vi "Label Targets AprilTagl.vi"(5 "Details":bool, 7 "Annotate":bool=TRUE, 9 "results":T1={"diameter points"={"first point"={"x"=0.0, "y"=0.0}, "projected point"={"x"=0.0, "y"=0.0}}, "normalized center"={"x"=0.0, "y"=0.0}, "Overall Score"=0.0, "Distance (ft)"=0.0, "Offset Angle"=0.0, "Tag corner points"=[], "Tag Center"={"X"=0.0, "Y"=0.0}, "Tag Yaw"=0.0, "Tag Pitch"=0.0, "Target Roll (deg)"=0.0, "AprilTag Number"=68} {"Tag Center"."Y" format="%0.2f"; "Tag Center"."X" format="%0.2f"}, 10 "Angle":dbl=53.2 format="%#_13g", 11 "Image in":T2) -> (3 "Image out":T2)   [LabVIEW 2023]
doc: "Draw scores near or on the particle and an ellipse around the target. Scores that are below the score threshold are drawn in red, above in green."
uses:
  <vilib>/vision/Image Controls.llb/IMAQ Image.ctl
  AprilTag Target Fields.ctl
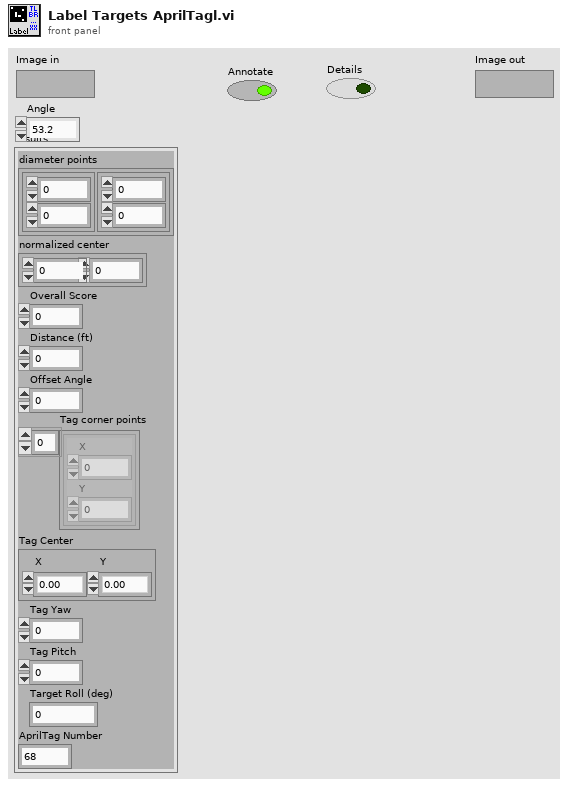
[diagram p1: front panel]
types:
  T1 = typedef "AprilTag Target Fields.ctl" = cluster{"diameter points":cluster{"first point":cluster{"x":dbl, "y":dbl}, "projected point":cluster{"x":dbl, "y":dbl}}, "normalized center":cluster{"x":dbl, "y":dbl}, "Overall Score":dbl, "Distance (ft)":dbl, "Offset Angle":dbl, "Tag corner points":cluster{"X":dbl, "Y":dbl}[], "Tag Center":cluster{"X":dbl, "Y":dbl}, "Tag Yaw":dbl, "Tag Pitch":dbl, "Target Roll (deg)":dbl, "AprilTag Number":i32}
  T2 = typedef "IMAQ Image.ctl" = refnum<image>
  T3 = cluster{"Desired Font (Application)":enum16{"User-specified Font", "Application Font", "System Font", "Dialog Font"}, "[User-specified Font]":cluster{"Font Name":string, "Size":i16, "Strikeout?":bool, "Italic?":bool, "Underline?":bool, "Outline?":bool, "Shadow?":bool, "Bold?":bool, "Rotation Angle":dbl}, "Horizontal Alignment":i16, "Vertical Alignment":i16}
  T4 = cluster{"first point":cluster{"x":dbl, "y":dbl}, "projected point":cluster{"x":dbl, "y":dbl}}
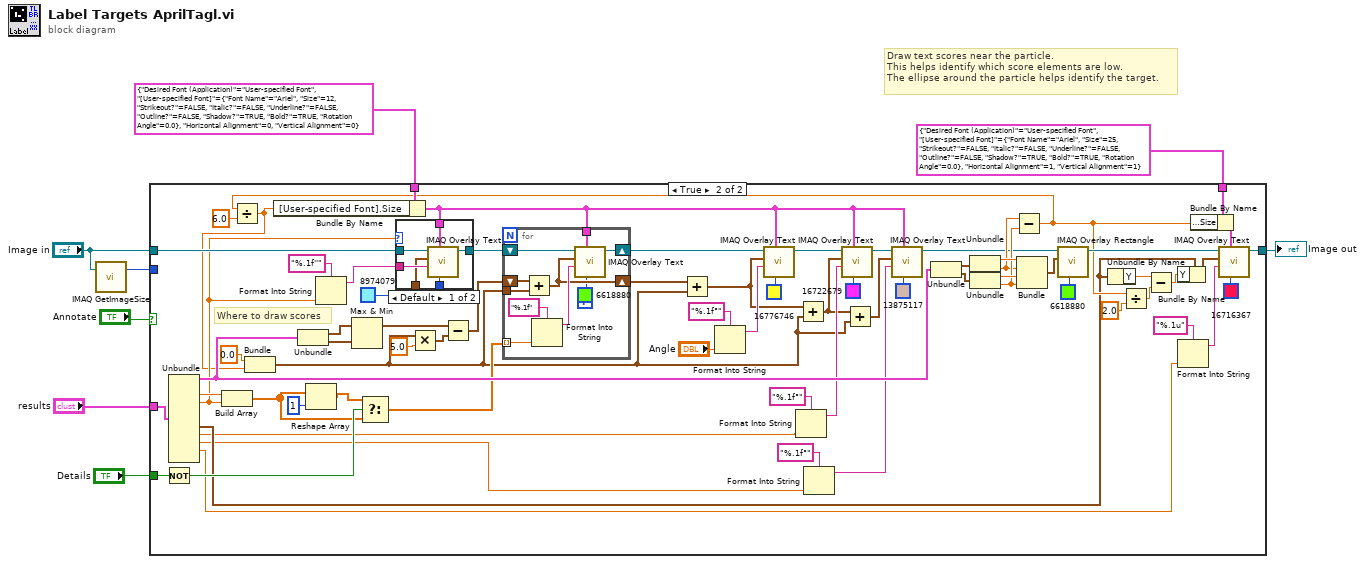
[diagram p0: block diagram]
diagram:
  # "Draw text scores near the particle.\nThis helps identify which score elements are low.\nThe ellipse around the particle helps identify the target."
  n1 = call "IMAQ GetImageSize"("Image"="Image in") -> ("Y Resolution"=w6:i32)  [unwired: 3 in, 2 out]
  n2 = case shown="True" "Annotate" {
    tunnel: [w9 w40] -> w8
    tunnel: "Image in" -> [w9 w79]
    tunnel: w6 -> [_ _]
    tunnel: "results" -> [_ w75]
    tunnel: "Details" -> [_ w66]
    tunnel: T3 {"Desired Font (Application)"=enum."User-specified Font", "[User-specified Font]"={"Font Name"="Ariel", "Size"=25, "Strikeout?"=FALSE, "Italic?"=FALSE, "Underline?"=FALSE, "Outline?"=FALSE, "Shadow?"=TRUE, "Bold?"=TRUE, "Rotation Angle"=0.0}, "Horizontal Alignment"=1, "Vertical Alignment"=1} ("Font, Size & Style") -> [_ w44]
    tunnel: T3 {"Desired Font (Application)"=enum."User-specified Font", "[User-specified Font]"={"Font Name"="Ariel", "Size"=12, "Strikeout?"=FALSE, "Italic?"=FALSE, "Underline?"=FALSE, "Outline?"=FALSE, "Shadow?"=TRUE, "Bold?"=TRUE, "Rotation Angle"=0.0}, "Horizontal Alignment"=0, "Vertical Alignment"=0} ("Font, Size & Style") -> [_ w26]
    frame False {
    }
    frame True {
      # "Where to draw scores"
      n3 = Not(x=w66) -> (.not. x?=w65:bool)
      n4 = Unbundle(w75) -> ("diameter points"=w70:T4, "Overall Score"=w59:dbl, "Distance (ft)"=w32:dbl, "Tag Center"=w13:cluster{"X":dbl, "Y":dbl}, "Tag Yaw"=w12:dbl, "Tag Pitch"=w11:dbl, "Target Roll (deg)"=w10:dbl)  [unwired: 4 out]
      n5 = Build Array(w59, w32) -> (w63:dbl[])
      n6 = Unbundle(w70) -> ("first point"=w72:cluster{"x":dbl, "y":dbl}, "projected point"=w73:cluster{"x":dbl, "y":dbl})
      n7 = Reshape Array(w63, 1) -> (w64:dbl[])
      n8 = Format Into String(format string="%.1f''", w32) -> (resulting string=w78:string)  [unwired: 2 in, 1 out]
      n9 = Max & Min(x=w72, y=w73) -> (max(x,y)=w51:cluster{"x":dbl, "y":dbl})  [unwired: 1 out]
      n10 = Select(t=w64, s=w65, f=w63) -> (s? t:f=w62:dbl[])
      n11 = Format Into String(format string="%.1f°", "Angle") -> (resulting string=w57:string)  [unwired: 2 in, 1 out]
      n12 = Format Into String(format string="%.1f°", w12) -> (resulting string=w31:string)  [unwired: 2 in, 1 out]
      n13 = Format Into String(format string="%.1f°", w11) -> (resulting string=w14:string)  [unwired: 2 in, 1 out]
      n14 = Unbundle(w70) -> ("first point"=w38:cluster{"x":dbl, "y":dbl}, "projected point"=w45:cluster{"x":dbl, "y":dbl})
      n15 = Unbundle(w38) -> ("x"=w69:dbl, "y"=w39:dbl)
      n16 = Unbundle(w45) -> ("x"=w68:dbl, "y"=w42:dbl)
      n17 = Subtract(x=w39, y=w42) -> (x-y=w25:dbl)
      n18 = Divide(x=w25, y=6.0) -> (x/y=w23:dbl)
      n19 = Bundle(0.0, w23) -> (w17:cluster{dbl, dbl})  [unwired: 1 in]
      n20 = Bundle By Name(cluster=w26, "[User-specified Font].Size"=w23) -> (w21:T3)
      n21 = Multiply(x=w17, y=5.0) -> (x*y=w50:cluster{dbl, dbl})
      n22 = Subtract(x=w51, y=w50) -> (x-y=w52:cluster{dbl, dbl})
      n23 = case shown="Default" w32 {
        tunnel: w79 -> [w95 w96]
        tunnel: w78 -> [w94 _]
        tunnel: w21 -> [w93 _]
        tunnel: [w92 w96] -> w74
        tunnel: w52 -> [w91 _]
        tunnel: u32 8974079 ("Color") -> [w90 _]
        frame Default {
          n24 = call "IMAQ Overlay Text"("Text Color (black)"=w90, "Font, Size & Style"=w93, "String"=w94, "Origin"=w91, "Image"=w95) -> ("Image Out"=w92:T2)  [unwired: 5 in, 1 out]
        }
        frame 0 {
        }
      }
      n25 = for {
        tunnel: w62 -> [w80] mode=indexing
        shift-right: [w86] -> w56
        shift-left: w74 -> [w87]
        tunnel: w21 -> [w85]
        shift-right: [w82] -> w53
        shift-left: w52 -> [w83]
        tunnel: w17 -> [w84]
        n26 = Add(x=w83, y=w84) -> (x+y=w82:cluster{dbl, dbl})
        n27 = Format Into String(format string="%.1f", w80) -> (resulting string=w88:string)  [unwired: 2 in, 1 out]
        n28 = call "IMAQ Overlay Text"("Text Color (black)"=u32 6618880 ("Color"), "Font, Size & Style"=w85, "String"=w88, "Origin"=w82, "Image"=w87) -> ("Image Out"=w86:T2)  [unwired: 5 in, 1 out]
      }
      n29 = Add(x=w53, y=w17) -> (x+y=w27:cluster{dbl, dbl})
      n30 = call "IMAQ Overlay Text"("Text Color (black)"=u32 16776746 ("Color"), "Font, Size & Style"=w21, "String"=w57, "Origin"=w27, "Image"=w56) -> ("Image Out"=w28:T2)  [unwired: 5 in, 1 out]
      n31 = Add(x=w27, y=w17) -> (x+y=w18:cluster{dbl, dbl})
      n32 = call "IMAQ Overlay Text"("Text Color (black)"=u32 16722679 ("Color"), "Font, Size & Style"=w21, "String"=w31, "Origin"=w18, "Image"=w28) -> ("Image Out"=w20:T2)  [unwired: 5 in, 1 out]
      n33 = Add(x=w18, y=w17) -> (x+y=w16:cluster{dbl, dbl})
      n34 = call "IMAQ Overlay Text"("Text Color (black)"=u32 13875117 ("Color"), "Font, Size & Style"=w21, "String"=w14, "Origin"=w16, "Image"=w20) -> ("Image Out"=w19:T2)  [unwired: 5 in, 1 out]
      n35 = Bundle("x"=w69, "y"=w39, "x"=w68, "y"=w42) -> (w67:cluster{"x":dbl, "y":dbl, "x":dbl, "y":dbl})  [unwired: 1 in]
      n36 = call "IMAQ Overlay Rectangle"("Color"=u32 6618880, "Rectangle"=w67, "Image"=w19) -> ("Image Out"=w41:T2)  [unwired: 7 in, 1 out]
      n37 = Unbundle By Name(w13) -> ("Y"=w36:dbl)
      n38 = Divide(x=w25, y=2.0) -> (x/y=w33:dbl)
      n39 = Subtract(x=w36, y=w33) -> (x-y=w35:dbl)
      n40 = Bundle By Name(cluster=w13, "Y"=w35) -> (w37:cluster{"X":dbl, "Y":dbl})
      n41 = Format Into String(format string="%.1u", w10) -> (resulting string=w47:string)  [unwired: 2 in, 1 out]
      n42 = Bundle By Name(cluster=w44, "[User-specified Font].Size"=w25) -> (w43:T3)
      n43 = call "IMAQ Overlay Text"("Text Color (black)"=u32 16716367 ("Color"), "Font, Size & Style"=w43, "String"=w47, "Origin"=w37, "Image"=w41) -> ("Image Out"=w40:T2)  [unwired: 5 in, 1 out]
    }
  }
  "Image out" <- w8
